vi "Start GNU OctaveNOVY.vi"(8 "error in":errorcluster, 10 "Octave binary directory":path, 11 "Working directory":path) -> (0 "error out":errorcluster, 1 "initial output":string, 2 "GNU Octave version":string, 3 "GOLPI ref. out":T1={"pipe handle"={"lv_proc.dll file path"=path "", "process instance handle"=[]}, "fast read timeout [ms]"=500, "fast read settle time [ms]"=10, "fast read to multiple [ms]"=1, "max elements per input line"=100, "slow read timeout [ms]"=500})   [LabVIEW 2013]
doc: "Starts the GNU Octave and sets the working directory. Returns GNU Octave version. Octave binary directory is the directory containing the 'octave.exe' executable file. Initial output is the informations printed after start on the screen by GNU Octave."
uses:
  Private/Type Definitions/GOLPI reference Type Def.ctl
  LV Process.lvlibp/Pipe Handle.ctl
  Private/Type Definitions/Custom Error Codes Enum Type Def.vi
  <vilib>/regexp/Match Regular Expression.xnode
  LV Process.lvlibp
  GOLPI library.lvlib
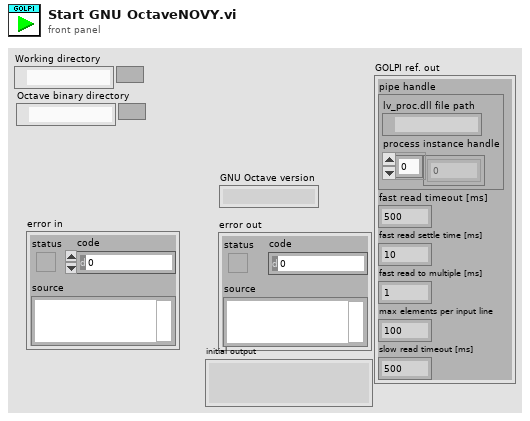
[diagram p1: front panel]
types:
  T1 = typedef "GOLPI library.lvlib/GOLPI reference Type Def.ctl" = cluster{"pipe handle":T2, "fast read timeout [ms]":u32, "fast read settle time [ms]":u32, "fast read to multiple [ms]":u32, "max elements per input line":u32, "slow read timeout [ms]":u32}
  T2 = typedef "LV Process.lvlibp/Pipe Handle.ctl" = cluster{"lv_proc.dll file path":path, "process instance handle":u32[]}
  T3 = typedef "GOLPI library.lvlib/Custom Error Codes Enum Type Def.vi" = enum16{"no error", "00 working directory PAR1 missing", "01 octave binary PAR1 missing", "02 octave report error PAR1", "03 empty output last cmd PAR1", "04 missing temporary file PAR1", "05 pwd PAR 1 not exist", "10 var PAR1 not string", "11 var PAR1 not num, scal, ~compl", "12 var PAR1 not num, scal, compl", "13 var PAR1 not num, vect, ~compl", "14 var PAR1 not num, vect, compl", "15 var PAR1 not num, mat, ~compl", "16 var PAR1 not num, mat, ~compl", "30 WARNING read timeout", "99 not finished"}
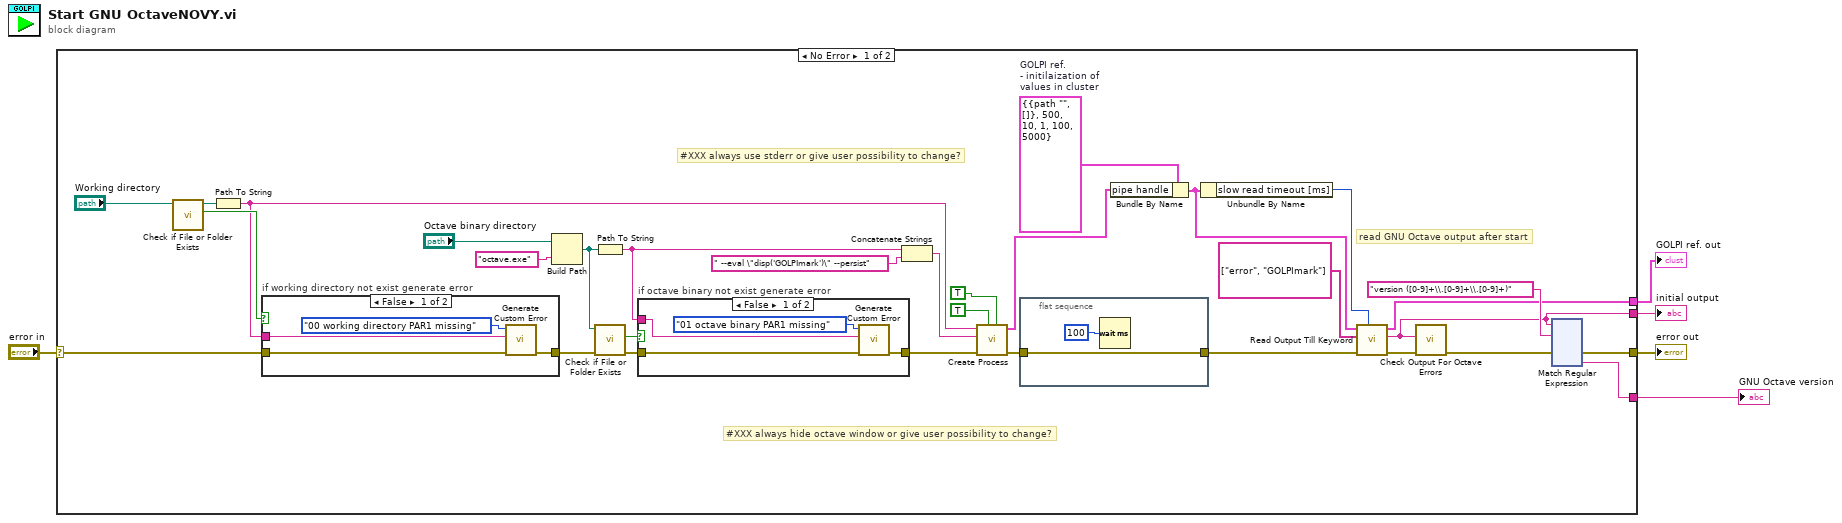
[diagram p0: block diagram]
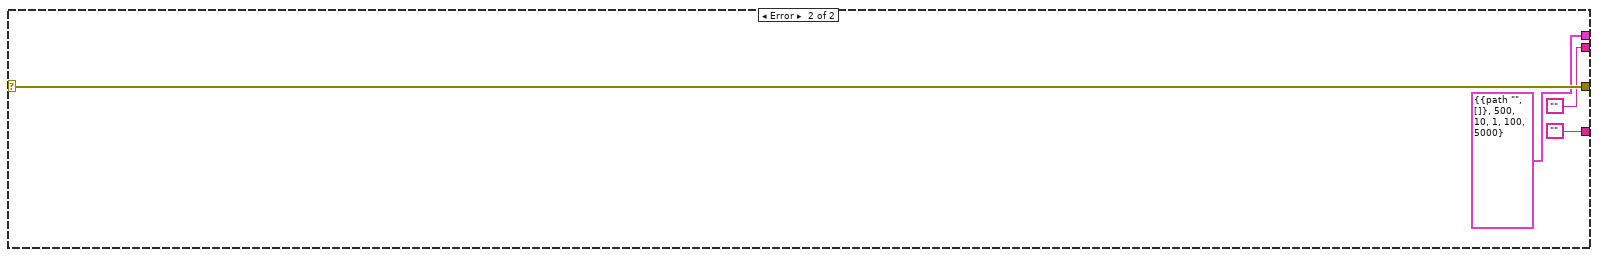
[diagram p4: hidden frame]
diagram:
  n1 = case shown="No Error" "error in" {
    selector: "error in" -> [w26 w168]
    tunnel: [w11 w168] -> w4
    tunnel: [w21 ""] -> w3
    tunnel: [w6 ""] -> w2
    tunnel: [w17 T1 {"pipe handle"={"lv_proc.dll file path"=path "", "process instance handle"=[]}, "fast read timeout [ms]"=500, "fast read settle time [ms]"=10, "fast read to multiple [ms]"=1, "max elements per input line"=100, "slow read timeout [ms]"=5000} ("GOLPI ref.")] -> w1
    frame No Error {
      w20 = T1 {"pipe handle"={"lv_proc.dll file path"=path "", "process instance handle"=[]}, "fast read timeout [ms]"=500, "fast read settle time [ms]"=10, "fast read to multiple [ms]"=1, "max elements per input line"=100, "slow read timeout [ms]"=5000}  # GOLPI ref. - initilaization of values in cluster
      # "read GNU Octave output after start"
      # "#XXX always hide octave window or give user possibility to change?"
      # "#XXX always use stderr or give user possibility to change?"
      n2 = call <vilib>:"Check if File or Folder Exists.vi"("path"="Working directory") -> ("file or folder exists?"=w32:bool, "dup path"=w33:path)  [unwired: 8 in, 1 out]
      n3 = Path To String(path=w33) -> (string=w31:string)
      n4 = case "if working directory not exist generate error" shown="False" w32 {
        tunnel: [w161 w164] -> w30
        tunnel: w26 -> [w160 w164]
        tunnel: w31 -> [w163 _]
        frame False {
          n5 = call "Generate Custom Error.vi"("error in"=w160, "PAR1"=w163, "GOLPI error"=Custom_Error_Codes_Enum_Type_Def.vi."00 working directory PAR1 missing" ("Enum")) -> ("error out"=w161:errorcluster)  [unwired: 8 in]
        }
        frame True {
        }
      }
      n6 = Build Path(base path="Octave binary directory", name or relative path="octave.exe" ("string")) -> (appended path=w25:path)
      n7 = Path To String(path=w25) -> (string=w14:string)
      n8 = call <vilib>:"Check if File or Folder Exists.vi"("error in (no error)"=w30, "path"=w25) -> ("error out"=w28:errorcluster, "file or folder exists?"=w29:bool)  [unwired: 7 in, 1 out]
      n9 = case "if octave binary not exist generate error" shown="False" w29 {
        tunnel: w28 -> [w156 w159]
        tunnel: [w155 w159] -> w27
        tunnel: w14 -> [w157 _]
        frame False {
          n10 = call "Generate Custom Error.vi"("error in"=w156, "PAR1"=w157, "GOLPI error"=Custom_Error_Codes_Enum_Type_Def.vi."01 octave binary PAR1 missing" ("Enum")) -> ("error out"=w155:errorcluster)  [unwired: 8 in]
        }
        frame True {
        }
      }
      n11 = Concatenate Strings(w14, " --eval \"disp('GOLPImark')\" --persist" ("string")) -> (w12:string)
      n12 = call "Create Process.vi"("use stderr (F)"=TRUE, "hide window (T)"=TRUE, "error in"=w27, "command"=w12, "working folder"=w31) -> ("error out"=w24:errorcluster, "pipe handle"=w19:T2)  [unwired: 5 in]
      n13 = flat-sequence {
        tunnel: [w153] -> w23
        tunnel: w24 -> [w153]
        frame #0 {
          n14 = Wait (ms)(milliseconds to wait=u32 100) -> ()  [unwired: 1 out]
        }
      }
      n15 = Bundle By Name(cluster=w20, "pipe handle"=w19) -> (w18:T1)
      n16 = Unbundle By Name(w18) -> ("slow read timeout [ms]"=w9:u32)
      n17 = call "Read Output Till Keyword.vi"("timeout [ms]"=w9, "error in"=w23, "keywords"=string[] ["error", "GOLPImark"], "GOLPI ref. in"=w18) -> ("error out"=w8:errorcluster, "read buffer"=w6:string, "GOLPI ref. out"=w17:T1)  [unwired: 4 in, 1 out]
      n18 = call "Check Output For Octave Errors.vi"("error in"=w8, "read buffer"=w6) -> ("error out"=w7:errorcluster)  [unwired: 9 in]
      n19 = xnode "Match Regular Expression"("input string"=w6, "regular expression"="version ([0-9]+\\.[0-9]+\\.[0-9]+)", "error in"=w7) -> ("error out"=w11:errorcluster, "submatch 1"=w21:string)  [unwired: 3 in, 4 out]
    }
    frame Error {
    }
  }
  "error out" <- w4
  "GNU Octave version" <- w3
  "initial output" <- w2
  "GOLPI ref. out" <- w1
